vi "fgv_PXI-5110_q-data.vi"(7 "cmd":T2, 8 "error in":errorcluster, 11 "data 2":T1={"Waveform(s)"=[{"relativeInitialX"=-1.5939337890625172e-05, "xIncrement"=1e-07, "wfm"=array[1000 elements]}], "Actual Record Length"=1000, "Actual Sample Rate"=10000000.0, "Auto Triggered"=FALSE}) -> (0 "error out":errorcluster, 3 "queue out":refnum<queue>)   [LabVIEW 2021]
uses:
  ctrl/5110_q.ctl
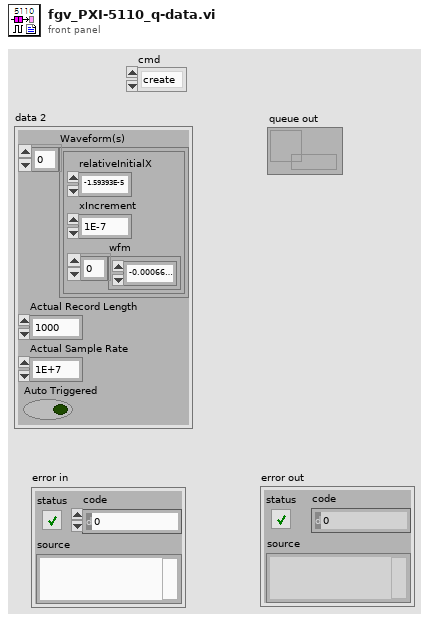
[diagram p1: front panel]
types:
  T1 = cluster{"Waveform(s)":cluster{"relativeInitialX":dbl, "xIncrement":dbl, "wfm":dbl[]}[], "Actual Record Length":i32, "Actual Sample Rate":dbl, "Auto Triggered":bool}
  T2 = typedef "5110_q.ctl" = enum16{"create", "read", "write", "close"}
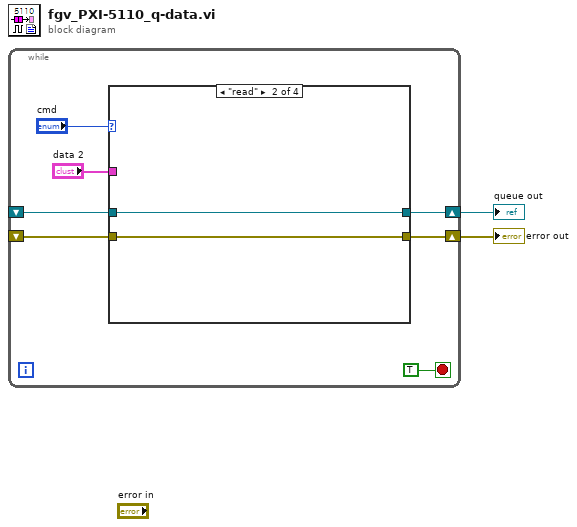
[diagram p0: block diagram]
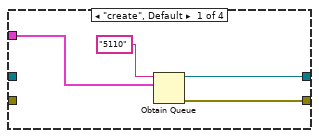
[diagram p2: hidden frame]
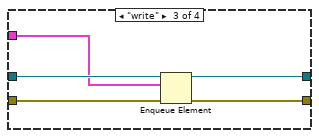
[diagram p3: hidden frame]
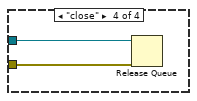
[diagram p4: hidden frame]
diagram:
  n1 = while {
    shift-right: [w7] -> w1
    shift-left: _ -> [w4]
    shift-right: [w6] -> w2
    shift-left: _ -> [w3]
    stop <- TRUE stop-if-true
    n2 = case shown="\"read\"" "cmd" {
      tunnel: [w13 w15 w17 _] -> w7
      tunnel: [w12 w14 w18 _] -> w6
      tunnel: "data 2" -> [w11 _ w16 _]
      tunnel: w4 -> [_ w15 w20 w22]
      tunnel: w3 -> [_ w14 w19 w21]
      frame "create", Default {
        n3 = Obtain Queue(name (unnamed)="5110", element data type=w11) -> (queue out=w13:refnum<queue>, error out=w12:errorcluster)  [unwired: 3 in, 1 out]
      }
      frame "read" {
      }
      frame "write" {
        n4 = Enqueue Element(queue=w20, element=w16, error in (no error)=w19) -> (queue out=w17:refnum<queue>, error out=w18:errorcluster)  [unwired: 1 in, 1 out]
      }
      frame "close" {
        n5 = Release Queue(queue=w22, error in (no error)=w21) -> ()  [unwired: 1 in, 3 out]
      }
    }
  }
  "error out" <- w2
  "queue out" <- w1
